vi "Delete LVClass from ProjectItem.vi"(7 "Delete Containing Folder?":bool, 8 "error in (no error)":errorcluster, 10 "LV Class Name":string, 11 "ProjectItem in":refnum<vi>) -> (0 "error out":errorcluster, 3 "ProjectItem out":refnum<vi>)   [LabVIEW 2019, in "gRPC Scripting Tools.lvlib"]
uses:
  gRPC Scripting Tools.lvlib
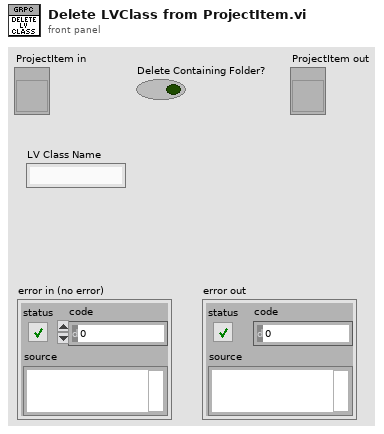
[diagram p1: front panel]
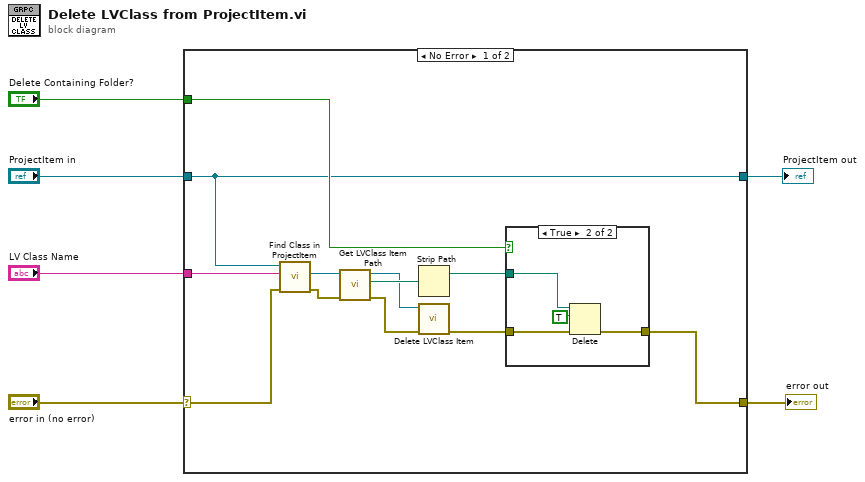
[diagram p0: block diagram]
diagram:
  n1 = case shown="No Error" "error in (no error)" {
    selector: "error in (no error)" -> [w8 w24]
    tunnel: [w17 w24] -> w6
    tunnel: "LV Class Name" -> [w10 _]
    tunnel: "ProjectItem in" -> [w7 w25]
    tunnel: "Delete Containing Folder?" -> [w9 _]
    tunnel: [w7 w25] -> w1
    frame No Error {
      n2 = call "Find Class in ProjectItem.vi"("error in (no error)"=w8, "Class Name"=w10, "ProjectItem in"=w7) -> ("error out"=w12:errorcluster, "LVClass out"=w11:refnum<vi>)  [unwired: 5 in, 2 out]
      n3 = call "Get LVClass Item Path.vi"("error in (no error)"=w12, "LVClassLibrary in"=w11) -> ("error out"=w14:errorcluster, "Path"=w18:path, "LVClassLibrary out"=w13:refnum<vi>)  [unwired: 7 in]
      n4 = Strip Path(path=w18) -> (stripped path=w16:path)  [unwired: 1 out]
      n5 = call "Delete LVClass Item.vi"("error in (no error)"=w14, "LVClassLibrary in"=w13) -> ("error out"=w15:errorcluster)  [unwired: 9 in]
      n6 = case shown="True" w9 {
        tunnel: [w19 w23] -> w17
        tunnel: w16 -> [_ w21]
        tunnel: w15 -> [w19 w20]
        frame False {
        }
        frame True {
          n7 = Delete(path (use dialog)=w21, entire hierarchy (F)=TRUE, error in=w20) -> (error out=w23:errorcluster)  [unwired: 2 in, 2 out]
        }
      }
    }
    frame Error {
    }
  }
  "error out" <- w6
  "ProjectItem out" <- w1
